vi "Make VI Param(Storage Info).vi"(1 "pStorageInfo":T1) -> (0 "Storage Info":T2)   [LabVIEW 8.6, in "Keyence LJ-V7000.lvlib"]
uses:
  Keyence LJ-V7000.lvlib
  Public/Clusters/Storage Info.ctl
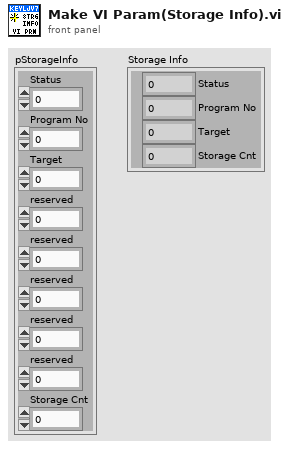
[diagram p1: front panel]
types:
  T1 = cluster{"Status":u8, "Program No":u8, "Target":u8, "reserved":u8, "reserved":u8, "reserved":u8, "reserved":u8, "reserved":u8, "Storage Cnt":u32}
  T2 = typedef "Keyence LJ-V7000.lvlib/Storage Info.ctl" = cluster{"Status":u8, "Program No":u8, "Target":u8, "Storage Cnt":u32}
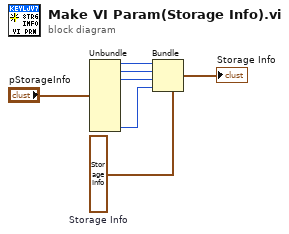
[diagram p0: block diagram]
diagram:
  w4 = T2 ?  # Storage Info
  n1 = Unbundle("pStorageInfo") -> ("Status"=w2:u8, "Program No"=w3:u8, "Target"=w5:u8, "Storage Cnt"=w6:u32)  [unwired: 5 out]
  n2 = Bundle(cluster=w4, "Status"=w2, "Program No"=w3, "Target"=w5, "Storage Cnt"=w6) -> (→"Storage Info":T2)
